vi "ClsGetOutputSignalIDs.vi"(8 "error in":errorcluster, 11 "Connection In":u32) -> (0 "error out":errorcluster, 2 "Singal IDs":i32[](array[numeric]), 3 "Connection Out":u32)   [LabVIEW 2015]
doc: "Get Output Signal IDs:\n\nUse this function for getting signal IDs for output. Any functions reading data out will have a format related to this signal IDs configuration. Please refer to the device manual for how signal IDs are defined in your device. Signal IDs smaller than 64 are used for CHRocodile 1 devices and Signal IDs greater or equal to 64 are used for CHRocodile 2 devices.\n\nConnection In[Input]: the connection handle which is initially created by Open Connection subVI.\n\nSignal IDs Out[Output]: The one dimensional signal IDs one dimensional array. Note that the order of the IDs here may be different from the input of the Set Output signals IDs subVI. The global signals will be ranked before the peak signals. \n\nConnection Out[Output]: the connection handle output which could be used for next subVI refering to the same connection."
uses:
  dependent dlls/CHRocodileDLL.dll
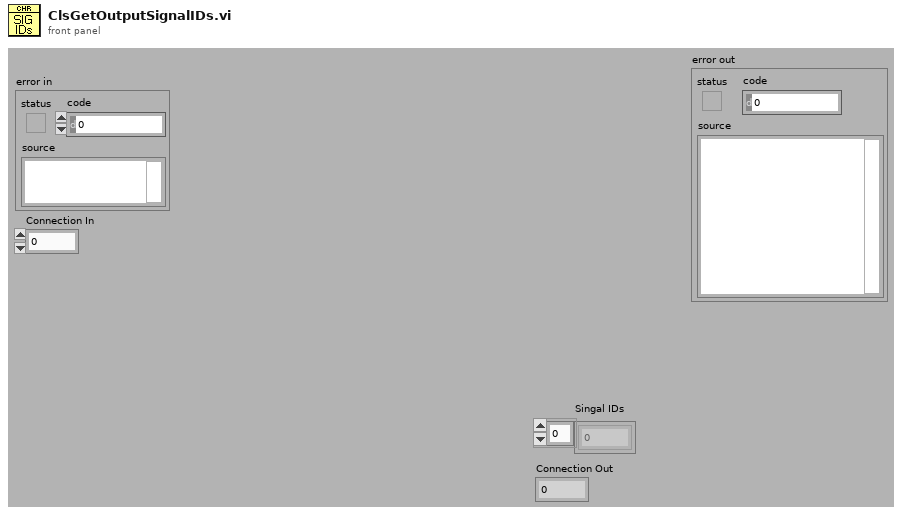
[diagram p1: front panel]
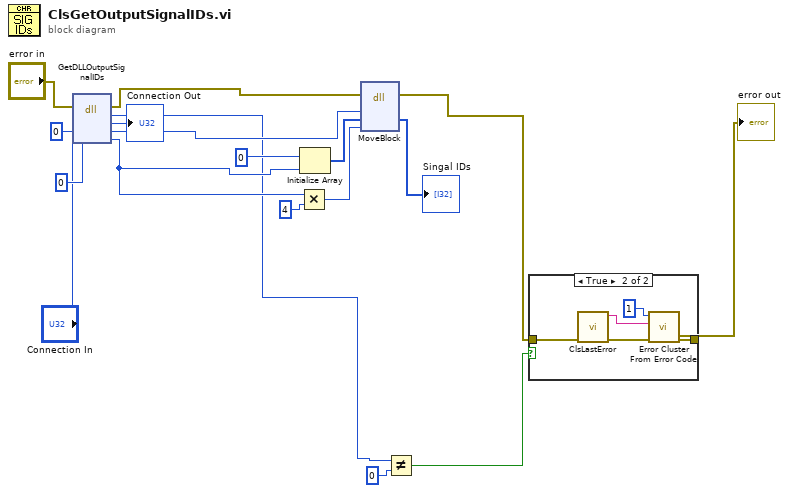
[diagram p0: block diagram]
diagram:
  n1 = dll-call lib="C:/Users/privat/Documents/ADP-SLA/Drop Impact Teststand/dependent dlls/CHRocodileDLL.*" fn="GetDLLOutputSignalIDs"(error in="error in", "_hConnection"="Connection In", "_pSignalIDbuffer"=i64 0 ("_pBuffer"), "_pSignalNr"=0 ("_nSampleNr")) -> (error out=w13:errorcluster, "return type"=w5:i32, "_hConnection"=→"Connection Out":u32, "_pSignalIDbuffer"=w12:i64, "_pSignalNr"=w11:i32)  [unwired: 2 in, 1 out]
  n2 = Multiply(x=w11, y=4) -> (x*y=w17:i32)
  n3 = Initialize Array(0, w11) -> (w15:i32[])
  n4 = dll-call lib="LabVIEW" fn="MoveBlock"(error in=w13, "Address(pointer)"=w12, "Destination"=w15, "Size"=w17) -> (error out=w3:errorcluster, "Destination"=→"Singal IDs":i32[])  [unwired: 5 in, 1 out]
  n5 = Not Equal?(x=w5, y=0) -> (x != y?=w4:bool)
  n6 = case shown="True" w4 {
    tunnel: [w19 w23] -> w2
    tunnel: w3 -> [w19 w20]
    frame False {
    }
    frame True {
      n7 = call "ClsLastError.vi"("error in (no error)"=w20) -> ("error out"=w21:errorcluster, "Error Message"=w22:string)  [unwired: 9 in]
      n8 = call <vilib>:"Error Cluster From Error Code.vi"("error in (no error)"=w21, "error message (\"\")"=w22, "error code (0)"=1) -> ("error out"=w23:errorcluster)  [unwired: 6 in]
    }
  }
  "error out" <- w2
